vi "Configure Temperature.vi"(8 "error in (no error)":errorcluster, 9 "Temperature Units (0: C)":i32(ring) items=["C", "F", "K"], 10 "Enable External Temperature Readings (F: Disable)":bool, 11 "VISA resource name":refnum<visa-resource-name>) -> (0 "error out":errorcluster, 3 "VISA resource name out":refnum<visa-resource-name>)   [LabVIEW 2016, in "Keithley 6517.lvlib"]
doc: "Configures the external temperature readings and the units for temperature readings (internal and external).\n\nNote:\nIt controls the temperature reading units for the multiple displays, buffer readings and readings sent out over the bus.\n\nThis VI is <B>NOT</B> compatible with model <B>6514</B>."
uses:
  <instrlib>/Keithley 6517/Keithley 6517.lvlib
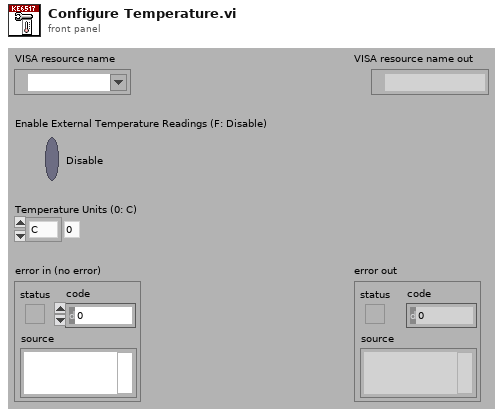
[diagram p1: front panel]
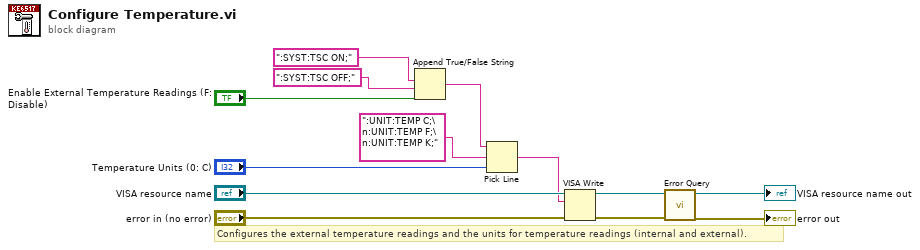
[diagram p0: block diagram]
diagram:
  # "Configures the external temperature readings and the units for temperature readings (internal and external)."
  n1 = Append True/False String(1:"Enable External Temperature Readings (F: Disable)", 2:":SYST:TSC OFF;", 3:":SYST:TSC ON;") -> (0:w2:string)  [unwired: 1 in]
  n2 = Pick Line(string ("")=w2, multi-line string=":UNIT:TEMP C;\n:UNIT:TEMP F;\n:UNIT:TEMP K;", line index="Temperature Units (0: C)") -> (output string=w1:string)
  n3 = VISA Write(VISA resource name="VISA resource name", write buffer=w1, error in (no error)="error in (no error)") -> (VISA resource name out=w8:refnum<visa-resource-name>, error out=w7:errorcluster)  [unwired: 1 out]
  n4 = call <instrlib>:"Error Query.vi"("error in (no error)"=w7, "VISA resource name"=w8) -> ("error out"=→"error out":errorcluster, "VISA resource name out"=→"VISA resource name out":refnum<visa-resource-name>)  [unwired: 6 in, 2 out]
